vi "Open.vi"(8 "error in (no error)":errorcluster caption="entrée d'erreur (pas d'erreur)", 11 "Class Camera IV3-500CA (Default) en entrée":refnum<class "Class Camera IV3-500CA.lvclass">) -> (0 "error out":errorcluster caption="sortie d'erreur", 3 "Class Camera IV3-500CA (Default) en Sortie":refnum<class "Class Camera IV3-500CA.lvclass">)   [LabVIEW 2020, in "Library Instrument & Equipement.lvlib" / "Library Camera.lvlib" / "Class Camera IV3-500CA.lvclass"]
uses:
  Class Camera IV3-500CA.lvclass
  C:/Users/ngarcin/OneDrive - Altyor/Standard TB/Class/Camera/Class Camera Pattern Matching (Default)/Class Pattern Matching (Default).lvclass
  Class Camera IV3-500CA.lvclass/Class Camera IV3-500CA.ctl
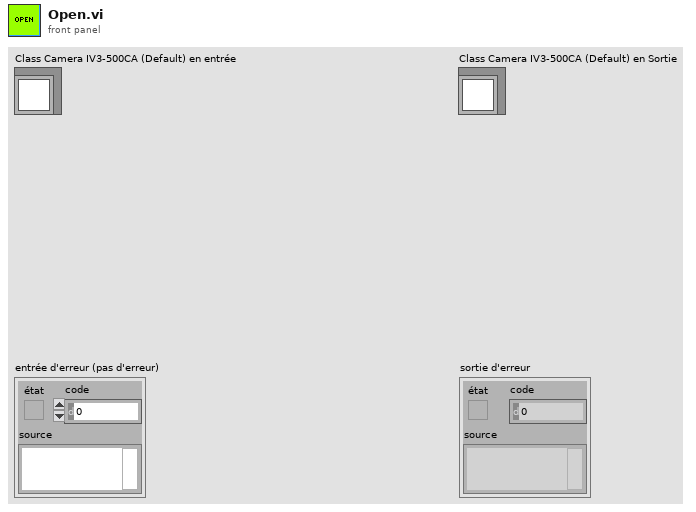
[diagram p1: front panel]
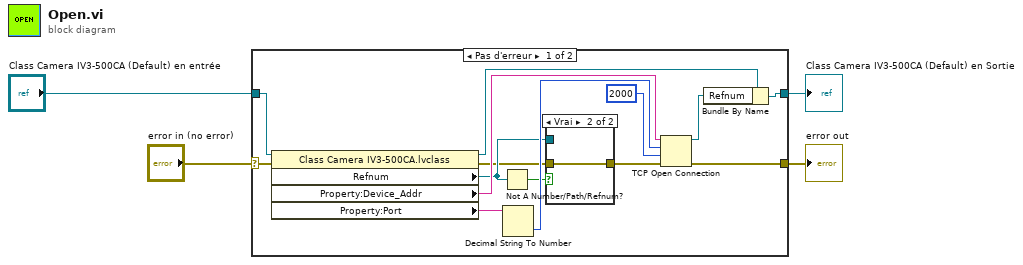
[diagram p0: block diagram]
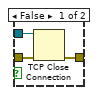
[diagram p2: hidden frame]
diagram:
  n1 = case shown="Pas d'erreur" "error in (no error)" {
    selector: "error in (no error)" -> [w11 w24]
    tunnel: [w18 w24] -> w3
    tunnel: [w16 w23] -> w1
    tunnel: "Class Camera IV3-500CA (Default) en entrée" -> [w17 w23]
    frame No Error {
      n2 = property class="Class Camera IV3-500CA.lvclass"(reference=w17, error in=w11) -> (reference out=w12:refnum<class "Class Camera IV3-500CA.lvclass">, error out=w5:errorcluster, "Refnum"=w7:refnum<k5>, "Property:Device_Addr"=w10:string, "Property:Port"=w9:string)
      n3 = Not A Number/Path/Refnum?(number/path/refnum=w7) -> (NaN/Path/Refnum?=w8:bool)
      n4 = Decimal String To Number(string=w9) -> (number=w13:i32)  [unwired: 2 in, 1 out]
      n5 = case shown="Vrai" w8 {
        tunnel: w7 -> [w21 _]
        tunnel: [w20 w22] -> w6
        tunnel: w5 -> [w19 w22]
        frame False {
          n6 = TCP Close Connection(connection ID=w21, error in (no error)=w19) -> (error out=w20:errorcluster)  [unwired: 1 in, 1 out]
        }
        frame True {
        }
      }
      n7 = TCP Open Connection(address=w10, remote port or service name=w13, timeout ms (60000)=2000 ("timeout en ms (60000)"), error in (no error)=w6) -> (connection ID=w15:refnum<k5>, error out=w18:errorcluster)  [unwired: 1 in]
      n8 = Bundle By Name(cluster=w12, "Refnum"=w15) -> (w16:refnum<class "Class Camera IV3-500CA.lvclass">)
    }
    frame Error {
    }
  }
  "error out" <- w3
  "Class Camera IV3-500CA (Default) en Sortie" <- w1
